vi "Read.vi"(8 "error in (no error)":errorcluster, 11 "Boolean in":refnum<class "UI-Bus_Waveform.lvclass">) -> (0 "error out":errorcluster, 2 "Value":T1, 3 "Boolean out":refnum<class "UI-Bus_Waveform.lvclass">)   [LabVIEW 2021, in "UI-Bus_Waveform.lvclass"]
doc: "Abstract Data Classes 2.1.1.13\nTim Streeter - TSA\nCopyright (c) 2025, TSA"
uses:
  UI-Bus_Waveform.lvclass
  Type.ctl
  UI-Bus_Waveform.lvclass/UI-Bus_Waveform.ctl
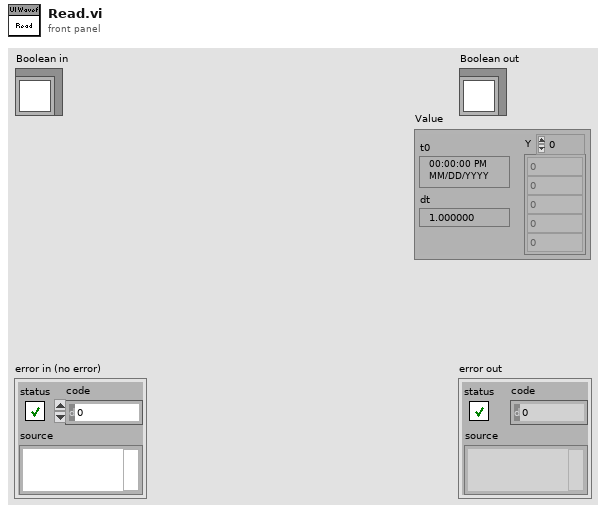
[diagram p1: front panel]
types:
  T1 = typedef "UI-Bus_Waveform.lvclass/Type.ctl" = waveform(dbl)
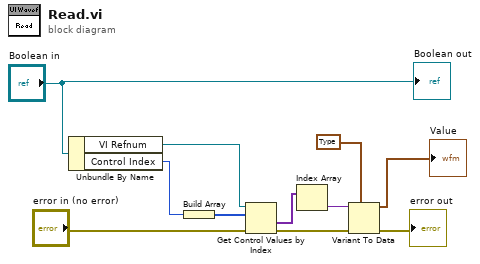
[diagram p0: block diagram]
diagram:
  n1 = Unbundle By Name("Boolean in") -> ("VI Refnum"=w9:refnum<vi>, "Control Index"=w8:i32)
  n2 = Build Array(w8) -> (w7:i32[])
  n3 = Get Control Values by Index(0:w9, 1:w7, 3:"error in (no error)") -> (10:w6:variant[], 11:w5:errorcluster)
  n4 = Index Array(array=w6) -> (element=w4:variant)  [unwired: 1 in]
  n5 = Variant To Data(error in=w5, type=T1 {"t0"=timestamp(0 s since 1904-01-01), "dt"=1.0, "Y"=[]} ("Value"), Variant=w4) -> (data=→"Value":T1, error out=→"error out":errorcluster)
  "Boolean out" <- "Boolean in"
